vi "Add Class.vi"(8 "error in (no error)":errorcluster, 10 "Class":string, 11 "Nav Route in":refnum<class "Nav Route.lvclass">) -> (0 "error out":errorcluster, 3 "Nav Route out":refnum<class "Nav Route.lvclass">)   [LabVIEW 2020, in "Volatus.lvlib" / "Nav Route.lvclass"]
uses:
  Nav Route.lvclass
  Nav Route.lvclass/Nav Route.ctl
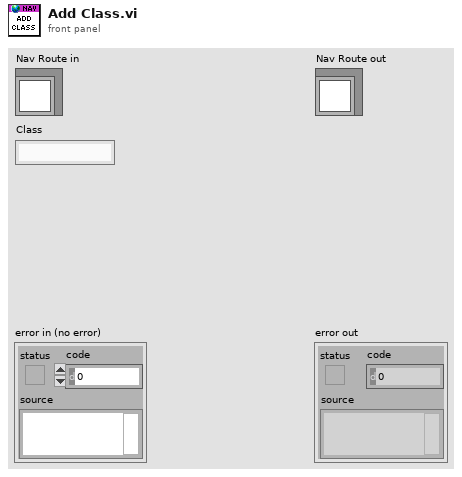
[diagram p1: front panel]
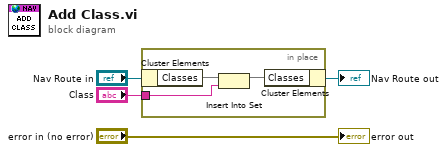
[diagram p0: block diagram]
diagram:
  n1 = in-place {
    in-place-border: "Class" -> [w6]
    n2 = in-place-cluster #1("Nav Route in") -> ("Classes"=w7:set{string})
    n3 = Insert Into Set(10:w6, 11:w7) -> (3:w5:set{string})  [unwired: 1 out]
    n4 = in-place-cluster #1("Classes"=w5) -> (→"Nav Route out":refnum<class "Nav Route.lvclass">)
  }
  "error out" <- "error in (no error)"
